vi "DriveModuleTrend.vi"(11 "Module":i32) -> ()   [LabVIEW 2025]
uses:
  frobotics-2025RobotCode/Dashboard-Testing/Dash_Globals.vi
  <vilib>/Rock Robotics/Network Tables/NT Read Number.vi
  <vilib>/Rock Robotics/Network Tables/NT Read Boolean.vi
panel:
  out "Const":bool
  out "Plant":bool
  out "PID_Done":bool
  out "CoStdDev":dbl format="%_8e"
  out "PvStdDev":dbl format="%_8e"
  out "Kd":dbl format="%_8e"
  out "Ki":dbl format="%_8e"
  out "Kp":dbl format="%_8e"
  out "Ka_StdDev":dbl format="%_8e"
  out "Ka_Calc":dbl format="%_8e"
  out "Ka_Done":bool
  out "Kv_SlowBck":dbl format="%_8e"
  out "Kv_SlowFwd":dbl format="%_8e"
  out "Kv_FastFwd":dbl format="%_8e"
  out "Swerve Mod":i32 format="%11.0f"
  out "Waveform Chart":T1(graph)
  out "Abs Angle Deg":dbl format="%11.1f"
  out "Dist Ft":dbl format="%11.2f"
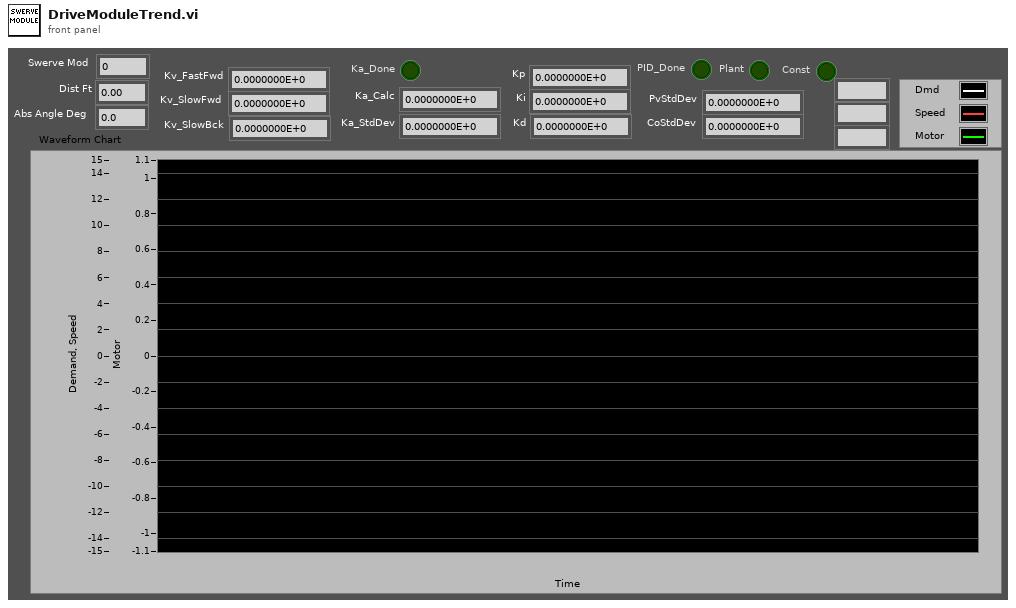
[diagram p1: front panel]
types:
  T1 = cluster{"TravSpdDmdFPS":dbl, "TravSpeedFPS":dbl, "TravMotDmd":dbl}
  T2 = enum8{"Tele-Op Disabled", "Tele-Op Enabled", "Auto Disabled", "Auto Enabled", "Test Disabled", "Test Enabled", "Disconnected", "No Code", "E-Stop"}
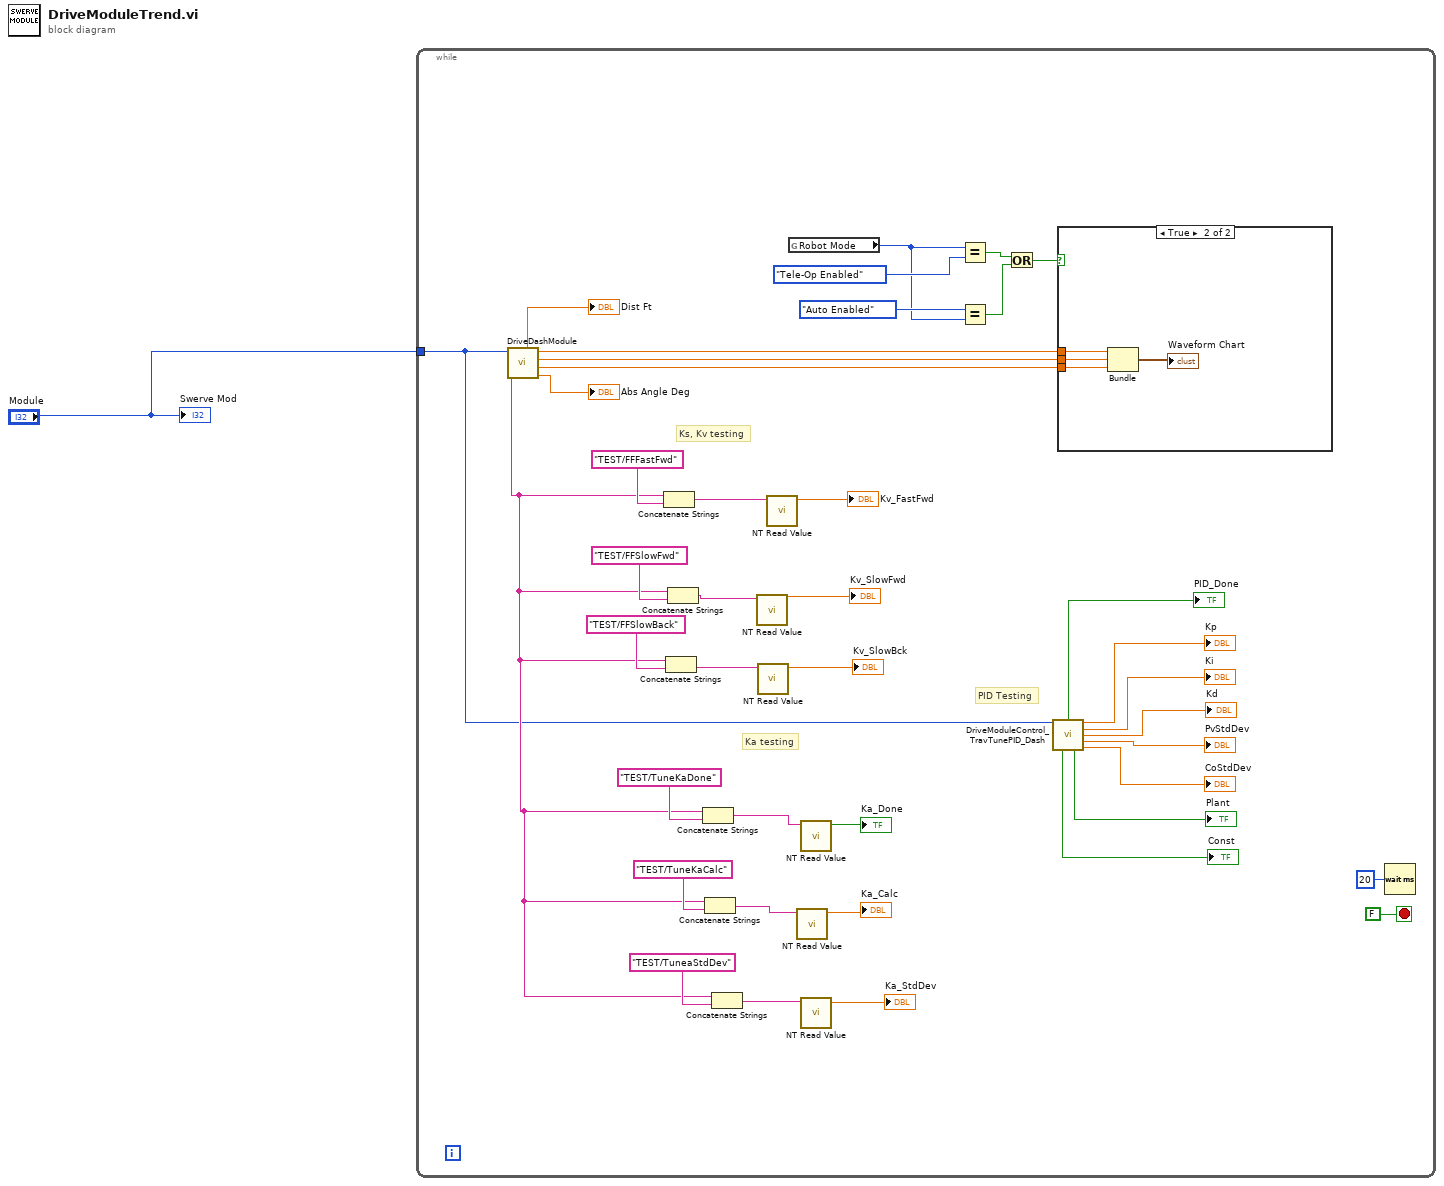
[diagram p0: block diagram]
diagram:
  n1 = while {
    tunnel: "Module" -> [w8]
    stop <- FALSE stop-if-true
    # "PID Testing"
    # "Ka testing"
    # "Ks, Kv testing"
    n2 = call "DriveDashModule.vi"("Module"=w8) -> ("SpinAbsPosDeg"=→"Abs Angle Deg":dbl, "TravMotDmd"=w38:dbl, "TravSpeedFPS"=w39:dbl, "TravSpdDmdFPS"=w40:dbl, "TravDistFt"=→"Dist Ft":dbl, "Prefix"=w17:string)  [unwired: 5 in]
    n3 = Concatenate Strings(w17, "TEST/FFFastFwd" ("refnum name")) -> (w34:string)
    n4 = Concatenate Strings(w17, "TEST/FFSlowBack" ("refnum name")) -> (w30:string)
    n5 = Concatenate Strings(w17, "TEST/FFSlowFwd" ("refnum name")) -> (w31:string)
    n6 = Concatenate Strings(w17, "TEST/TuneKaDone" ("name")) -> (w23:string)
    n7 = Concatenate Strings(w17, "TEST/TuneKaCalc" ("name")) -> (w22:string)
    n8 = Concatenate Strings(w17, "TEST/TuneaStdDev" ("name")) -> (w21:string)
    n9 = call-poly <vilib>:"NT Read Value.vi"("name"=w31) -> ("value"=→"Kv_SlowFwd":dbl)  [unwired: 8 in, 2 out]
    n10 = call-poly <vilib>:"NT Read Value.vi"("name"=w30) -> ("value"=→"Kv_SlowBck":dbl)  [unwired: 8 in, 2 out]
    n11 = call-poly <vilib>:"NT Read Value.vi"("name"=w34) -> ("value"=→"Kv_FastFwd":dbl)  [unwired: 8 in, 2 out]
    n12 = global read "Dash_Globals.vi" "Robot Mode"() -> (w5:T2)
    n13 = call-poly <vilib>:"NT Read Value.vi"("name"=w22) -> ("value"=→"Ka_Calc":dbl)  [unwired: 8 in, 2 out]
    n14 = call-poly <vilib>:"NT Read Value.vi"("name"=w23) -> ("value"=→"Ka_Done":bool)  [unwired: 8 in, 2 out]
    n15 = call-poly <vilib>:"NT Read Value.vi"("name"=w21) -> ("value"=→"Ka_StdDev":dbl)  [unwired: 8 in, 2 out]
    n16 = Equal?(x=w5, y=T2."Tele-Op Enabled") -> (x = y?=w4:bool)
    n17 = Equal?(x=T2."Auto Enabled" ("y"), y=w5) -> (x = y?=w3:bool)
    n18 = Or(x=w4, y=w3) -> (x .or. y?=w2:bool)
    n19 = call "DriveModuleControl_TravTunePID_Dash.vi"("Network Table Prefix"=w8) -> ("TestDone"=→"PID_Done":bool, "Kp"=→"Kp":dbl, "Ki"=→"Ki":dbl, "Kd"=→"Kd":dbl, "PvStdDev"=→"PvStdDev":dbl, "ConstDone"=→"Const":bool, "PlantDone"=→"Plant":bool, "CoStdDev"=→"CoStdDev":dbl)  [unwired: 5 in, 2 out]
    n20 = case shown="True" w2 {
      tunnel: w40 -> [_ w46]
      tunnel: w39 -> [_ w45]
      tunnel: w38 -> [_ w44]
      frame False {
      }
      frame True {
        n21 = Bundle("TravSpdDmdFPS"=w46, "TravSpeedFPS"=w45, "TravMotDmd"=w44) -> (→"Waveform Chart":T1)  [unwired: 1 in]
      }
    }
    n22 = Wait (ms)(milliseconds to wait=u32 20) -> ()  [unwired: 1 out]
  }
  "Swerve Mod" <- "Module"
